vi "testAppBuilder_fpga.vi"() -> ()   [LabVIEW 2014]
uses:
  <vilib>/rvi/Emulation/niFpgaGetClockAttributes.vi
  <vilib>/rvi/Emulation/niFpgaSctlEmulationGetInTimedLoop.vi
  <vilib>/rvi/Emulation/niFpgaEmulationReportErrorSimple.vi
  <vilib>/rvi/Emulation/niFpgaCriticalErrorInLSC.vi
panel:
  in  "input_STOP":bool
  out "output_num":i16
  in  "input_num":i16
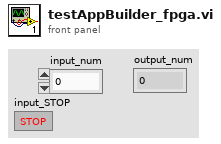
[diagram p1: front panel]
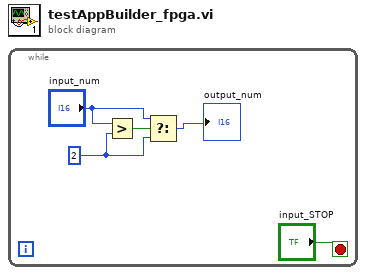
[diagram p0: block diagram]
diagram:
  n1 = while {
    stop <- "input_STOP" stop-if-true
    w4 = i16 2 ("y")
    n2 = Greater?(x="input_num", y=w4) -> (0:w5:bool)
    n3 = Select(t="input_num", s=w5, f=w4) -> (s? t:f=→"output_num":i16)
  }
